vi "pruebas.vi"() -> ()   [LabVIEW 2020]
panel:
  out "x*y":dbl[](array[numeric])
  out "output array":dbl[][](array[numeric])
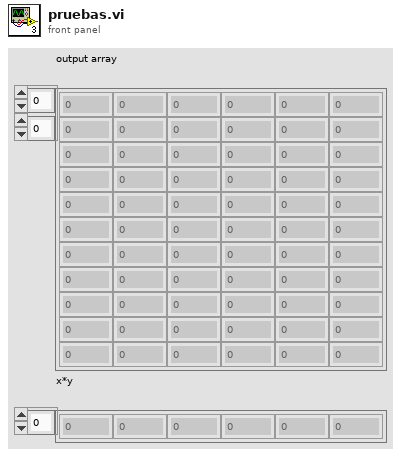
[diagram p1: front panel]
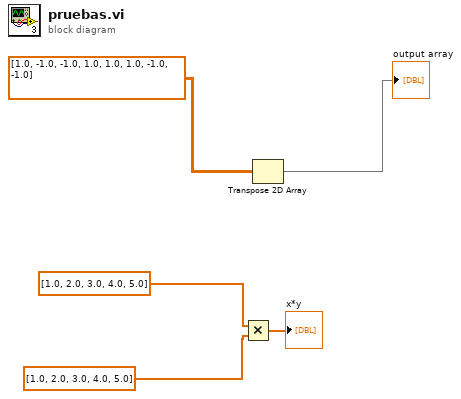
[diagram p0: block diagram]
diagram:
  n1 = Multiply(x=dbl[] [1.0, 2.0, 3.0, 4.0, 5.0], y=dbl[] [1.0, 2.0, 3.0, 4.0, 5.0]) -> (x*y=→"x*y":dbl[])
  n2 = Transpose 2D Array(2D array=dbl[][] [[1.0, -1.0, -1.0, 1.0], [1.0, 1.0, -1.0, -1.0]]) -> (transposed array=→"output array":dbl[][])
